vi "ecc register error code n2e.vi"(1 "number":u32 format="%0d") -> (0 "enum":T1)   [LabVIEW 2024, in "atsj peakcan basic.lvlib"]
uses:
  ecc register error code.ctl
  atsj peakcan basic.lvlib
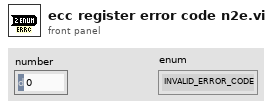
[diagram p1: front panel]
types:
  T1 = typedef "atsj peakcan basic.lvlib/ecc register error code.ctl" = enum8{"INVALID_ERROR_CODE", "COUNTERS_UPDATE", "BIT_ERROR", "FORM_ERROR", "STUFF_ERROR", "OTHER_ERROR"}
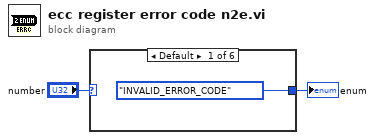
[diagram p0: block diagram]
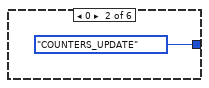
[diagram p2: hidden frame]
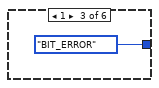
[diagram p3: hidden frame]
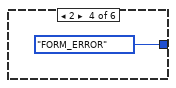
[diagram p4: hidden frame]
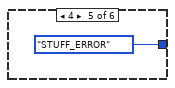
[diagram p5: hidden frame]
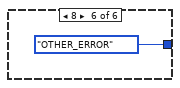
[diagram p6: hidden frame]
diagram:
  n1 = case shown="Default" "number" {
    tunnel: [ecc_register_error_code."INVALID_ERROR_CODE" ecc_register_error_code."COUNTERS_UPDATE" ecc_register_error_code."BIT_ERROR" ecc_register_error_code."FORM_ERROR" ecc_register_error_code."STUFF_ERROR" ecc_register_error_code."OTHER_ERROR"] -> w1
    frame Default {
    }
    frame 0 {
    }
    frame 1 {
    }
    frame 2 {
    }
    frame 4 {
    }
    frame 8 {
    }
  }
  "enum" <- w1
